vi "StitchingModeLabspec6_KJM.vi"(9 "Data In":dbl[][][](array[numeric])) -> (2 "Simple Stitched Data Out":dbl[][](array[numeric]))   [LabVIEW 2020]
doc: "Stitches spectra based on simple cut-off modus."
uses:
  4c98e68f-fed8-44bd-a6f6-c5aabdf5d44d.vi
  <vilib>/numeric/Random Number (Range) U64.vi
  7ace7b3b-a852-4920-82e1-5223555fe086.vi
panel:
  out "deleted portion 3":dbl[](array[numeric])
  out "deleted portion 2":dbl[](array[numeric])
  out "transposed array":dbl[][](array[numeric])
  out "spectrum 2, before/overlap?":dbl[][](array[numeric])
  out "spectrum , before/overlap? 1":dbl[][](array[numeric])
  out "spectrum 1, before/overlap?":dbl[][](array[numeric])
  out "spectrum 1, before/overlap?":dbl[][](array[numeric])
  out "overlap end":dbl
  out "overlap start":dbl
  out "appended array 2":dbl[][](array[numeric])
  out "Empty Array 2":dbl[][][](array[numeric])
  out "Linear Stitch Data Out":dbl[][](array[numeric])
  out "Array 5":dbl[](array[numeric])
  out "s? t:f 2":dbl
  out "s? t:f":dbl
  out "Array 4":bool[](array[boolean])
  out "Array 3":dbl[](array[numeric])
  out "Array 2":dbl[](array[numeric])
  out "Array":dbl[](array[numeric])
  out "appended array 8":dbl[](array[numeric])
  out "appended array 6":dbl[](array[numeric])
  out "appended array 5":dbl[][](array[numeric])
  out "x1":dbl[](array[numeric])
  out "x2":dbl[](array[numeric])
  out "appended array 4":dbl[][](array[numeric])
  out "appended array 3":dbl[][](array[numeric])
  out "appended array":dbl[][][](array[numeric])
  out "y2":dbl[][](array[numeric])
  out "y1":dbl[][](array[numeric])
  out "deleted portion":dbl[][](array[numeric])
  out "array w/ subset deleted":dbl[][](array[numeric])
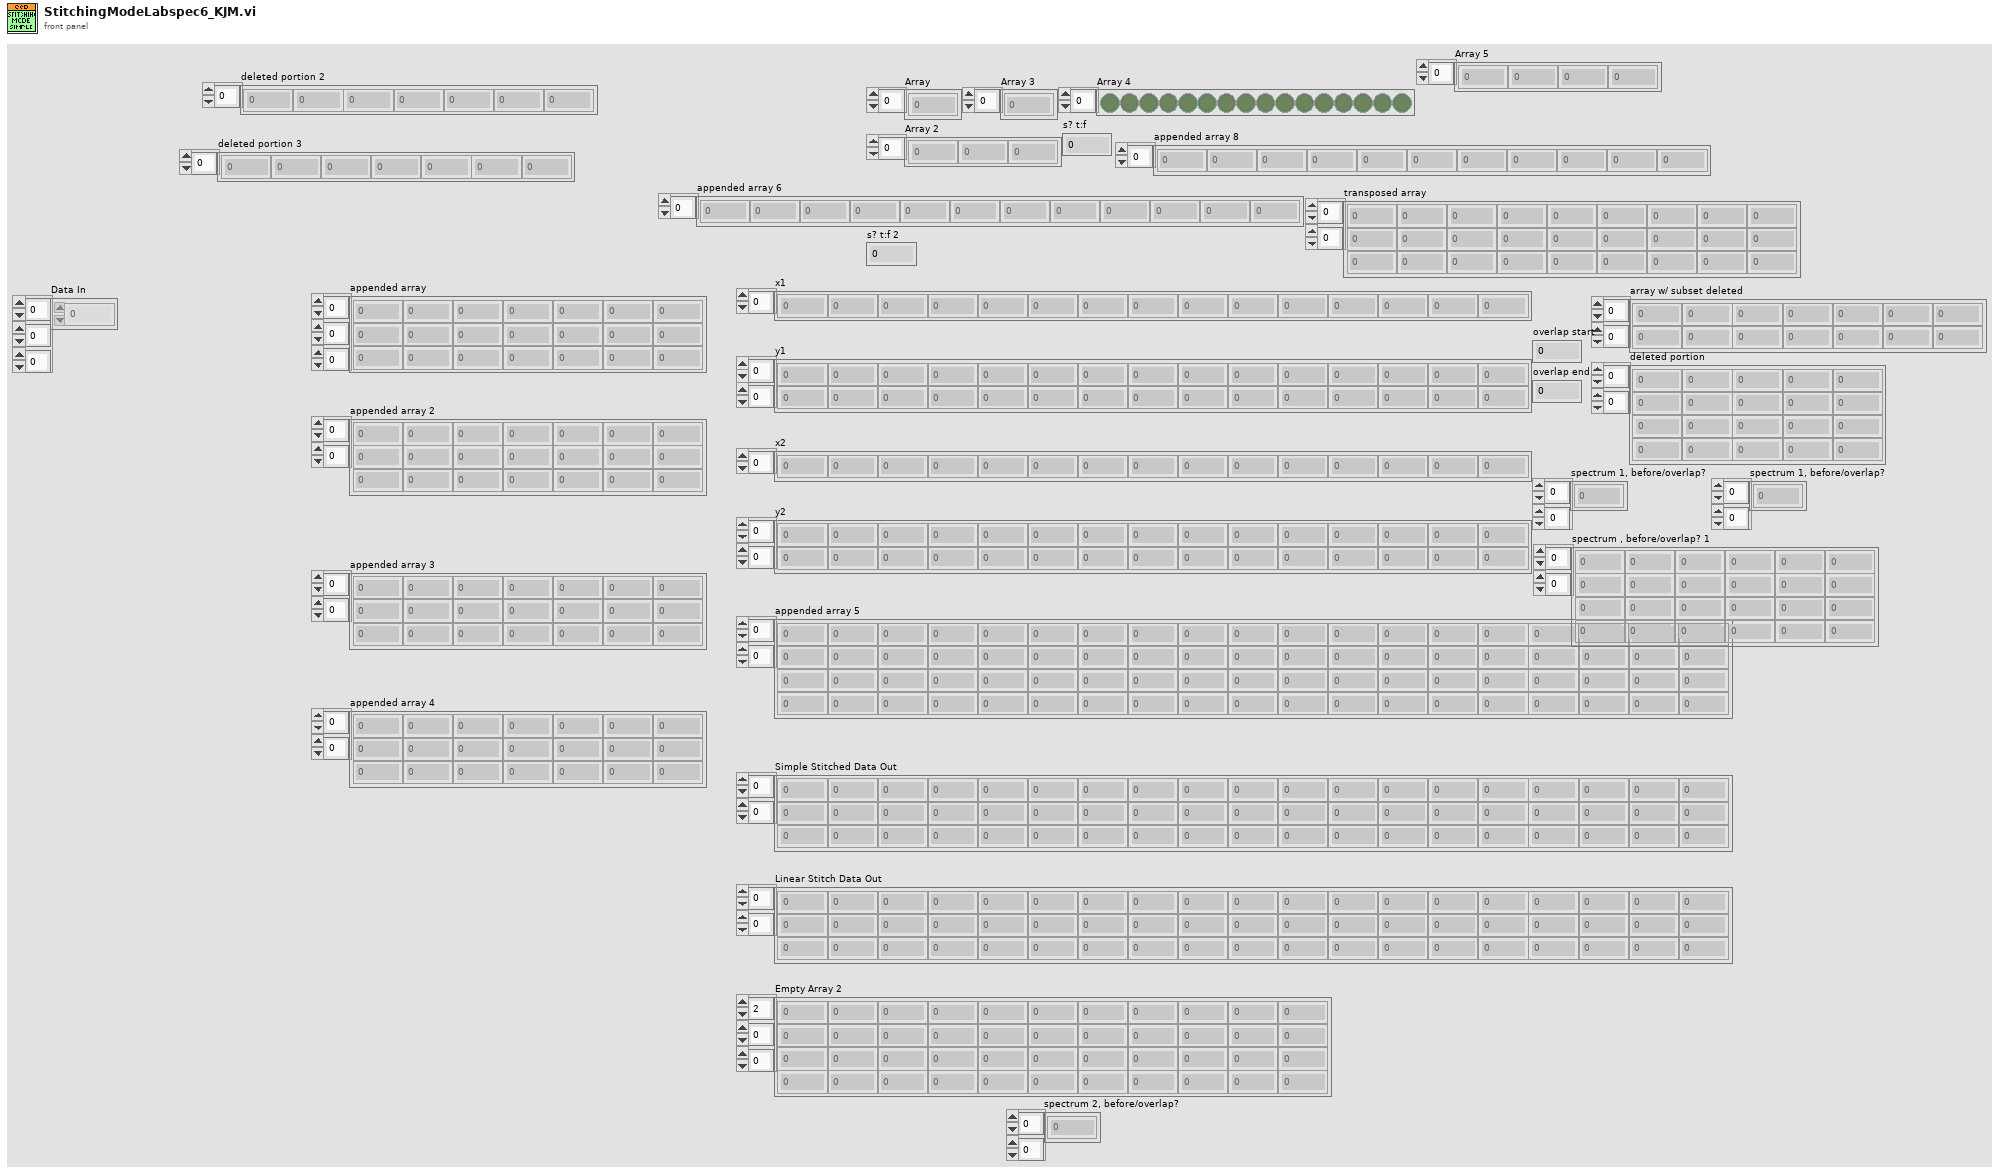
[diagram p1: front panel]
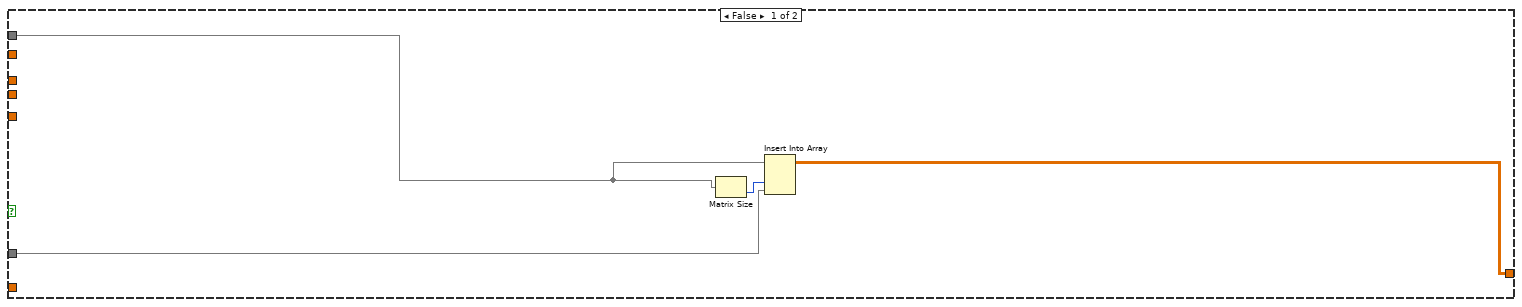
[diagram p3: hidden frame]
diagram:
  # "/* x1 with mask 1 */"
  n1 = while {
    stop <- TRUE stop-if-true
    # "/* Expects a 3D array where:\n1) Each page is a separate CCD acquisition.\n2) The first row of each page is the x data (typically wavelengths)\n3) The rest of the rows are intensity data at each wavelength  */"
    n2 = for {
      N: 6 -> [_]
      tunnel: [w34] -> w16 mode=indexing
      tunnel: [w38] -> w15 mode=indexing
      i -> [w37]
      n3 = Random Number (0-1)() -> (number: 0 to 1=w35:dbl)
      n4 = call-poly <vilib>:"Random Number (Range).vi"("lower bound (0)"=u64 800, "upper bound (100)"=u64 1000) -> ("number"=w38:u64)  [unwired: 9 in]
      n5 = Compound Arithmetic op=ADD(w35, 400 ("x"), w37) -> (w34:dbl)
    }
    n6 = for {
      N: 6 -> [_]
      tunnel: [w30] -> w12 mode=indexing
      tunnel: [w31] -> w11 mode=indexing
      i -> [w29]
      n7 = Random Number (0-1)() -> (number: 0 to 1=w27:dbl)
      n8 = call-poly <vilib>:"Random Number (Range).vi"("lower bound (0)"=u64 800, "upper bound (100)"=u64 1000) -> ("number"=w31:u64)  [unwired: 9 in]
      n9 = Compound Arithmetic op=ADD(w27, 402.0, w29) -> (w30:dbl)
    }
    n10 = for {
      N: 6 -> [_]
      tunnel: [w23] -> w9 mode=indexing
      tunnel: [w24] -> w8 mode=indexing
      i -> [w22]
      n11 = Random Number (0-1)() -> (number: 0 to 1=w20:dbl)
      n12 = call-poly <vilib>:"Random Number (Range).vi"("lower bound (0)"=u64 800, "upper bound (100)"=u64 1000) -> ("number"=w24:u64)  [unwired: 9 in]
      n13 = Compound Arithmetic op=ADD(w20, 408.1, w22) -> (w23:dbl)
    }
    n14 = Build Array(w16, w15) -> (w14:dbl[][])
    "appended array 2" <- w14
    n15 = Build Array(w12, w11) -> (w7:dbl[][])
    "appended array 3" <- w7
    n16 = Build Array(w9, w8) -> (→"appended array 4":dbl[][])
    n17 = Build Array(w14, w7) -> (w5:dbl[][][])
    "appended array" <- w5
    n18 = for {
      tunnel: w5 -> [w54] mode=indexing
      shift-right: [w61] -> w19
      shift-left: dbl[][] [] ("Empty Array") -> [w59]
      shift-right: [w41] -> w3
      shift-left: dbl[][] [] ("Empty Array") -> [w51]
      tunnel: [w44] -> _
      tunnel: [w41] -> w1 mode=indexing
      # "/* Sort by first row \n(x data) */"
      n19 = Empty Array?(array=w59) -> (empty?=w60:bool)
      n20 = call "Sort 2D Array.vim"("index"=0, "dimension to index (column)"=1 ("index"), "2D array"=w54) -> ("sorted 2D array"=w53:dbl[][])  [unwired: 7 in, 1 out]
      n21 = Transpose 2D Array(2D array=w53) -> (transposed array=w58:dbl[][])
      n22 = for {
        tunnel: w58 -> [w71] mode=indexing
        tunnel: [w71] -> w57 mode=indexing if=w72
        # "/* Deletes columns with zero\nin their x data, caused by\nmistmatched data sizes */"
        n23 = Not Equal To 0?(x=w71) -> (x != 0?=w70:bool[])
        n24 = Or Array Elements(Boolean array=w70) -> (logical OR=w72:bool)
      }
      n25 = Transpose 2D Array(2D array=w57) -> (transposed array=w52:dbl[][])
      "transposed array" <- w52
      n26 = case shown="False" w60 {
        tunnel: [w105 w197] -> w61
        tunnel: w52 -> [w79 w197]
        tunnel: w59 -> [w88 _]
        tunnel: [w89 w197] -> w41
        tunnel: w51 -> [w78 _]
        frame False {
          # "/* spectrum 1 */"
          # "/* spectrum 2 */"
          # "/* Splits first spectrum into\ny1 (top) and x1 (bottom) */"
          # "/* Splits second spectrum into\ny2 (top) and x2 (bottom) */"
          # "/* labspec */"
          # "/* overlap end */"
          # "/* overlap start */"
          # "/* Concatenates data \ncolumn-wise */"
          # "/* Checks for x data overlap \nin spectra/images */"
          n27 = Delete From Array(array=w79, index (row)=0) -> (deleted portion=w98:dbl[], array with subset deleted=w97:dbl[][])  [unwired: 2 in]
          "y2" <- w97
          "x2" <- w98
          n28 = Delete From Array(array=w78, index (row)=0) -> (deleted portion=w99:dbl[], array with subset deleted=w96:dbl[][])  [unwired: 2 in]
          "y1" <- w96
          "x1" <- w99
          n29 = Delete From Array(array=w79, index (row)=0) -> (deleted portion=w75:dbl[])  [unwired: 2 in, 1 out]
          "deleted portion 2" <- w75
          n30 = Delete From Array(array=w78, index (row)=0) -> (deleted portion=w76:dbl[])  [unwired: 2 in, 1 out]
          n31 = Index Array(array=w88, index (row)=0) -> (element=w110:dbl[])  [unwired: 1 in]
          n32 = Index Array(array=w79, index (row)=0) -> (element=w112:dbl[])  [unwired: 1 in]
          n33 = Array Max & Min(array=w99) -> (max value=w92:dbl, min value=w95:dbl)  [unwired: 2 out]
          n34 = Array Max & Min(array=w98) -> (max value=w91:dbl, min value=w94:dbl)  [unwired: 2 out]
          n35 = Delete From Array(array=w75) -> (deleted portion=w74:dbl)  [unwired: 2 in, 1 out]
          n36 = Delete From Array(array=w76) -> (deleted portion=w73:dbl)  [unwired: 2 in, 1 out]
          n37 = Index Array(array=w75, index=0) -> (element=w83:dbl)
          n38 = Index Array(array=w76, index=0) -> (element=w82:dbl)
          n39 = Array Max & Min(array=w110) -> (max value=w109:dbl)  [unwired: 3 out]
          n40 = Array Max & Min(array=w112) -> (min value=w108:dbl)  [unwired: 3 out]
          n41 = Less Or Equal?(x=w92, y=w91) -> (x <= y?=w90:bool)
          n42 = Greater Or Equal?(x=w92, y=w94) -> (x >= y?=w102:bool)
          n43 = Greater Or Equal?(x=w95, y=w94) -> (x >= y?=w93:bool)
          n44 = Max & Min(x=w74, y=w73) -> (min(x,y)=w77:dbl)  [unwired: 1 out]
          "overlap end" <- w77
          n45 = Max & Min(x=w83, y=w82) -> (max(x,y)=w80:dbl)  [unwired: 1 out]
          "overlap start" <- w80
          n46 = Greater Or Equal?(x=w109, y=w108) -> (x >= y?=w107:bool)
          n47 = Select(t=w92, s=w90, f=w91) -> (s? t:f=w100:dbl)
          "s? t:f" <- w100
          n48 = Select(t=w95, s=w93, f=w94) -> (s? t:f=w101:dbl)
          "s? t:f 2" <- w101
          n49 = Greater?(x=w77, y=w80) -> (0:w81:bool)
          n50 = case shown="True" w102 {
            tunnel: w101 -> [_ w158]
            tunnel: w100 -> [_ w157]
            tunnel: w99 -> [_ w156]
            tunnel: w98 -> [_ w159]
            tunnel: w97 -> [_ w141]
            tunnel: w96 -> [_ w152]
            tunnel: [w133 w137] -> w89
            tunnel: w78 -> [w135 _]
            tunnel: w79 -> [w134 _]
            frame False {
              n51 = Matrix Size(0:w135) -> (2:w136:i32)  [unwired: 1 out]
              n52 = Insert Into Array(array=w135, index (col)=w136, new element=w134) -> (w133:dbl[][])  [unwired: 1 in]
            }
            frame True {
              # "/* y1 with mask 1 */"
              # "/* x1 with ~mask1 */"
              # "/* y2 with ~mask 2 */"
              # "/* x1 with mask 1 */"
              # "/* y2 with mask 2 */"
              # "/* x2 with ~mask 2 */"
              # "/* x2 with mask 2 */"
              n53 = Index Array(array=w152, index (row)=0) -> (element=w153:dbl[])  [unwired: 1 in]
              n54 = for {
                tunnel: w156 -> [w180] mode=indexing
                tunnel: w158 -> [w182]
                tunnel: w157 -> [w181]
                tunnel: [w180] -> w149 mode=indexing if=w177
                tunnel: [w180] -> w150 mode=indexing if=w178
                tunnel: [w179] -> w154 mode=indexing if=w177
                tunnel: w153 -> [w179] mode=indexing
                tunnel: [w179] -> w147 mode=indexing if=w178
                tunnel: [w177] -> w138 mode=indexing
                n55 = Greater Or Equal?(x=w180, y=w182) -> (x >= y?=w184:bool)
                n56 = Less Or Equal?(x=w180, y=w181) -> (x <= y?=w183:bool)
                n57 = And(x=w184, y=w183) -> (x .and. y?=w177:bool)
                n58 = Not(x=w177) -> (.not. x?=w178:bool)
              }
              "Array" <- w150
              "Array 2" <- w149
              "Array 4" <- w138
              "Array 5" <- w149
              n59 = Index Array(array=w141, index (row)=0) -> (element=w140:dbl[])  [unwired: 1 in]
              n60 = for {
                tunnel: w159 -> [w172] mode=indexing
                tunnel: w158 -> [w174]
                tunnel: w157 -> [w173]
                tunnel: [w172] -> w155 mode=indexing if=w171
                tunnel: [w172] -> w148 mode=indexing if=w169
                tunnel: [w170] -> w139 mode=indexing if=w171
                tunnel: w140 -> [w170] mode=indexing
                tunnel: [w170] -> w145 mode=indexing if=w169
                # "/* y2 with mask 2 */"
                n61 = Greater Or Equal?(x=w172, y=w174) -> (x >= y?=w176:bool)
                n62 = Less Or Equal?(x=w172, y=w173) -> (x <= y?=w175:bool)
                n63 = And(x=w176, y=w175) -> (x .and. y?=w171:bool)
                n64 = Not(x=w171) -> (.not. x?=w169:bool)
              }
              "Array 3" <- w148
              n65 = for {
                tunnel: w155 -> [w167]
                tunnel: w149 -> [w164] mode=indexing
                tunnel: w154 -> [w165] mode=indexing
                tunnel: [w161] -> w146 mode=indexing
                tunnel: w139 -> [w160]
                n66 = Threshold 1D Array(2:w164, 3:w167) -> (0:w168:dbl)  [unwired: 1 in]
                n67 = Interpolate 1D Array(1:w168, 2:w160) -> (0:w166:dbl)
                n68 = Add(x=w165, y=w166) -> (x+y=w163:dbl)
                n69 = Divide(x=w163, y=2.0) -> (x/y=w161:dbl)
              }
              n70 = Build Array (concatenate)(w150, w149, w148) -> (w144:dbl[])
              "appended array 6" <- w144
              n71 = Build Array (concatenate)(w147, w146, w145) -> (w143:dbl[])
              "appended array 8" <- w143
              n72 = Build Array(w144, w143) -> (w137:dbl[][])
              "appended array 5" <- w137
            }
          }
          n73 = case shown="True" w81 {
            tunnel: w80 -> [_ w130]
            tunnel: w79 -> [_ w117]
            tunnel: w78 -> [_ w128]
            tunnel: w77 -> [_ w115]
            tunnel: w76 -> [_ w129]
            tunnel: w75 -> [_ w116]
            frame False {
            }
            frame True {
              n74 = Threshold 1D Array(2:w130, 3:w129) -> (0:w132:dbl)  [unwired: 1 in]
              n75 = Threshold 1D Array(2:w115, 3:w116) -> (0:w123:dbl)  [unwired: 1 in]
              n76 = Round Toward +Infinity(x=w132) -> (ceil(x): smallest int >= x=w124:dbl)
              n77 = Matrix Size(0:w128) -> (2:w131:i32)  [unwired: 1 out]
              n78 = Round Toward +Infinity(x=w123) -> (ceil(x): smallest int >= x=w118:dbl)
              n79 = Subtract(x=w131, y=w124) -> (x-y=w125:dbl)
              n80 = Matrix Size(0:w117) -> (2:w122:i32)  [unwired: 1 out]
              n81 = Delete From Array(array=w128, length=w125, index (col)=w124) -> (deleted portion=→"spectrum 1, before/overlap?":dbl[][], array with subset deleted=→"spectrum 1, before/overlap?":dbl[][])  [unwired: 1 in]
              n82 = Subtract(x=w122, y=w118) -> (x-y=w119:dbl)
              n83 = Delete From Array(array=w117, length=w119, index (col)=w118) -> (deleted portion=→"spectrum 2, before/overlap?":dbl[][], array with subset deleted=→"spectrum , before/overlap? 1":dbl[][])  [unwired: 1 in]
            }
          }
          n84 = case shown="True" w107 {
            tunnel: w88 -> [w185 w191]
            tunnel: [w185 w195] -> w106
            tunnel: w108 -> [_ w194]
            tunnel: w110 -> [_ w193]
            frame False {
              # "/* Passes previous data if \nthere is no overlap */"
            }
            frame True {
              # "/* Trims columns of previous \ndata after the overlap starts  */"
              n85 = Matrix Size(0:w191) -> (2:w190:i32)  [unwired: 1 out]
              n86 = Threshold 1D Array(2:w194, 3:w193) -> (0:w192:dbl)  [unwired: 1 in]
              n87 = Round Toward +Infinity(x=w192) -> (ceil(x): smallest int >= x=w188:dbl)
              n88 = Subtract(x=w190, y=w188) -> (x-y=w189:dbl)
              n89 = Delete From Array(array=w191, length=w189, index (col)=w188) -> (deleted portion=→"deleted portion":dbl[][], array with subset deleted=→"array w/ subset deleted":dbl[][])  [unwired: 1 in]
              n90 = Array Subset(array=w191, index (col)=0 ("index"), length (col)=w188) -> (w195:dbl[][])  [unwired: 2 in]
            }
          }
          n91 = Matrix Size(0:w106) -> (2:w111:i32)  [unwired: 1 out]
          n92 = Insert Into Array(array=w106, index (col)=w111, new element=w79) -> (w105:dbl[][])  [unwired: 1 in]
        }
        frame True {
          # "/* This case will run on the first loop iteration */"
        }
      }
      n93 = call "Sort 2D Array.vim"("index"=0, "dimension to index (column)"=1 ("index"), "2D array"=w41) -> ("sorted 2D array"=w48:dbl[][])  [unwired: 7 in, 1 out]
      n94 = Index Array(array=w48, index (row)=0) -> (element=w43:dbl[])  [unwired: 1 in]
      n95 = Array Size(array=w43) -> (size(s)=w42:i32)
      n96 = Index Array(array=w41, index (row)=0) -> (element=w45:dbl[])  [unwired: 1 in]
      n97 = while {
        tunnel: w43 -> [w69] mode=indexing
        tunnel: w45 -> [w68] mode=indexing
        tunnel: [w63] -> w44
        tunnel: [w65] -> _
        tunnel: w42 -> [w65]
        i -> [w66]
        stop <- w62 stop-if-true
        n98 = Greater?(x=w66, y=w65) -> (0:w64:bool)
        n99 = Equal?(x=w68, y=w69) -> (x = y?=w67:bool)
        n100 = Not(x=w67) -> (.not. x?=w63:bool)
        n101 = Or(x=w64, y=w63) -> (x .or. y?=w62:bool)
      }
    }
    "Simple Stitched Data Out" <- w19
    "Linear Stitch Data Out" <- w3
    "Empty Array 2" <- w1
  }
